vi "TLight.vi"(10 "Array":bool[](array[boolean])) -> (2 "Array 2":u32[](array[colorbox]))   [LabVIEW 2019]
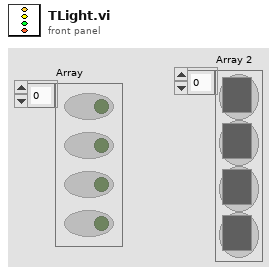
[diagram p1: front panel]
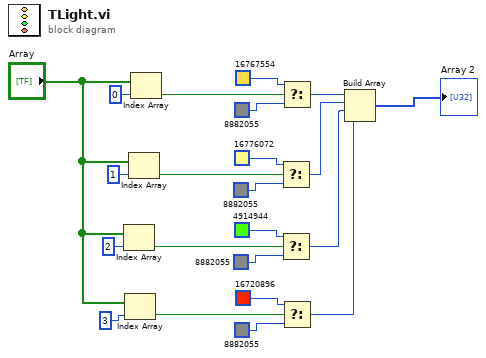
[diagram p0: block diagram]
diagram:
  n1 = Index Array(array="Array", index=2) -> (element=w12:bool)
  n2 = Index Array(array="Array", index=3) -> (element=w2:bool)
  n3 = Index Array(array="Array", index=1) -> (element=w11:bool)
  n4 = Index Array(array="Array", index=0) -> (element=w13:bool)
  n5 = Select(t=u32 16776072 ("Red 2"), s=w11, f=u32 8882055 ("Red 2")) -> (s? t:f=w8:u32)
  n6 = Select(t=u32 4914944 ("Red 2"), s=w12, f=u32 8882055 ("Red 2")) -> (s? t:f=w7:u32)
  n7 = Select(t=u32 16767554 ("Red 2"), s=w13, f=u32 8882055 ("Red 2")) -> (s? t:f=w10:u32)
  n8 = Select(t=u32 16720896 ("Red 2"), s=w2, f=u32 8882055 ("Red 2")) -> (s? t:f=w1:u32)
  n9 = Build Array(w10, w8, w7, w1) -> (→"Array 2":u32[])
